vi "BRig_dataExp_T_Timeout.vi"() -> (2 "output_T_Timeout":i32)   [LabVIEW 2014]
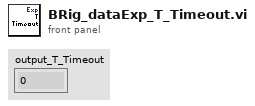
[diagram p1: front panel]
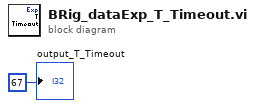
[diagram p0: block diagram]
diagram:
  "output_T_Timeout" <- 67 ("output_iBlock")
